vi "TDMS Filename.vi"(9 "Serial Number":string, 10 "Model Number":string, 11 "Test Type":string) -> (3 "Filename":string)   [LabVIEW 2011]
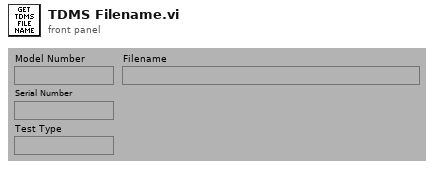
[diagram p1: front panel]
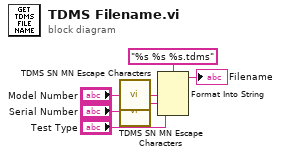
[diagram p0: block diagram]
diagram:
  n1 = call "TDMS SN MN Escape Characters.vi"("string"="Model Number") -> ("url-encoded string"=w4:string)
  n2 = call "TDMS SN MN Escape Characters.vi"("string"="Serial Number") -> ("url-encoded string"=w2:string)
  n3 = Format Into String(format string="%s %s %s.tdms", w4, w2, "Test Type") -> (resulting string=→"Filename":string)  [unwired: 2 in, 1 out]
